vi "Demo.vi"() -> ()   [LabVIEW 2013]
panel:
  out "Adc 2":dbl[](graph)
  out "Adc 1":dbl[](graph)
  in  "Numeric 2":i32=1
  in  "Frequency":i32
  in  "Samples":u16=1
  out "Device info":string
  in  "VISA resource name":refnum<visa-resource-name>="ASRL2::INSTR"
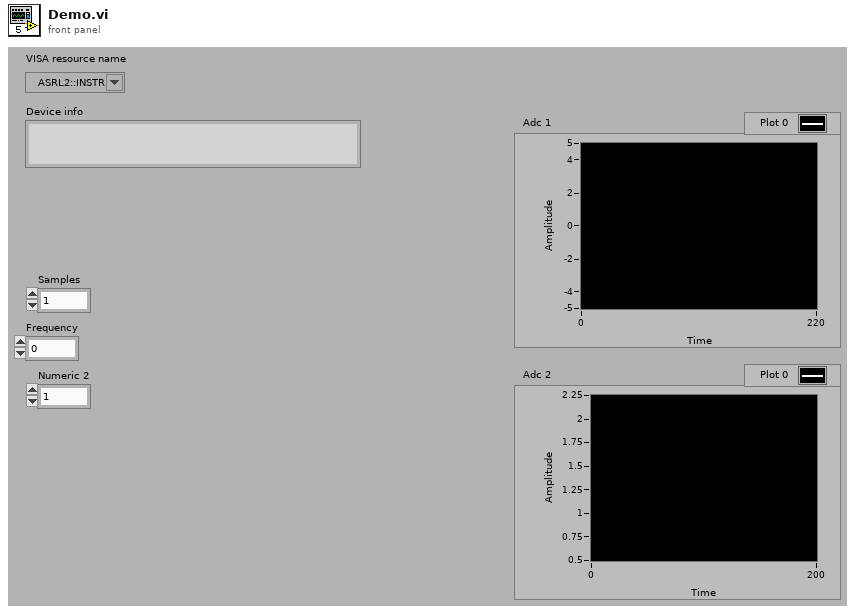
[diagram p1: front panel]
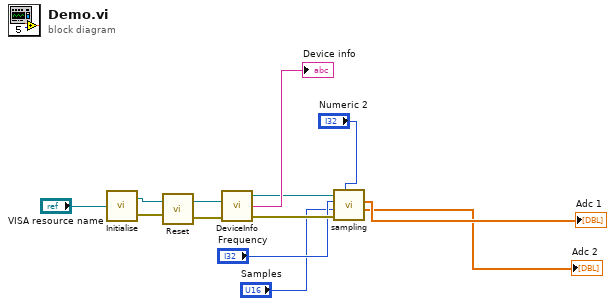
[diagram p0: block diagram]
diagram:
  n1 = call "Initialise.vi"("VISA resource name"="VISA resource name") -> ("Duplicate VISA resource name"=w11:refnum<visa-resource-name>, "Error out"=w10:errorcluster)
  n2 = call "Reset.vi"("error in (no error)"=w10, "VISA resource name"=w11) -> ("Error out"=w9:errorcluster, "Duplicate VISA resource name"=w8:refnum<visa-resource-name>)
  n3 = call "DeviceInfo.vi"("VISA resource name"=w8, "Error in (no error)"=w9) -> ("VISA resource name out"=w7:refnum<visa-resource-name>, "Device info"=→"Device info":string, "Error out"=w6:errorcluster)
  n4 = call "sampling.vi"("Active channels"="Numeric 2", "Error in (no error)"=w6, "Samples"="Samples", "Frequency"="Frequency", "VISA resource name"=w7) -> ("Adc 2"=→"Adc 2":dbl[], "Adc 1"=→"Adc 1":dbl[])  [unwired: 2 out]
